vi "dischage_check.vi"(8 "error in":errorcluster) -> (0 "error out":errorcluster)   [LabVIEW 2019]
uses:
  hw-control.ctl
  _ctrl/BP4610_cmd.ctl
  _ctrl/DSP_action.ctl
  _ctrl/init-w-close.ctl
  f7c2fc01-ab73-4381-998f-938b9d5f35cd.vi
  bbb9578e-c01f-4956-a005-e59b9cab9503.vi
  27d873ac-d62a-41d9-9b50-5c3ef5b223c2.vi
  d86a43f2-1348-4437-a8b3-b480884b10c3.vi
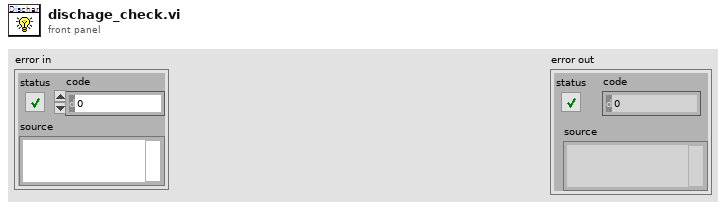
[diagram p1: front panel]
types:
  T1 = typedef "init-w-close.ctl" = enum16{"open", "init", "write", "close"}
  T2 = typedef "DSP_action.ctl" = enum16{"False", "cont", "on", "off", "discont", "protection", "protection_seq", "preread", "level_seq", "level_m", "read", "stop", "exit"}
  T3 = typedef "BP4610_cmd.ctl" = enum16{"open", "read", "set", "set_seq", "limit", "limit_seq", "output on", "output off", "close"}
  T4 = typedef "hw-control.ctl" = enum16{"DL950 ready", "DL950 clear", "DL950 trigger", "DL950 read", "DL950 read seq", "DL950 Tsingle query", "AO 12v", "AO wave", "AO 0v", "relay all-off", "Discharge check", "Discharge", "Relay1", "Relay2", "Relay3", "Relay4", "Relay5", "Relay6", "BP4610 onoff", "BP4610 set", "DSP1500 set", "DSP1500 onoff"}
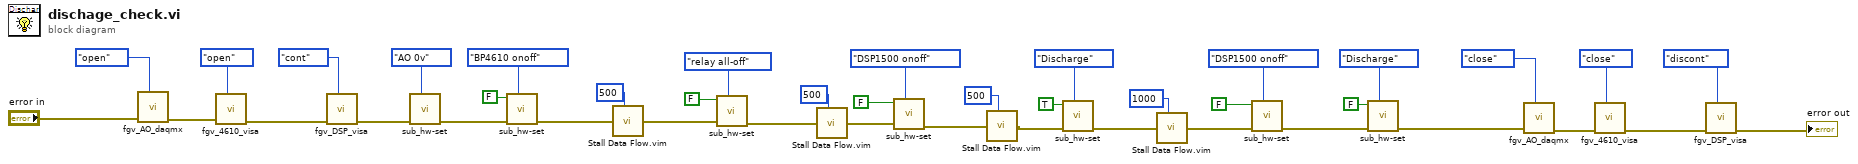
[diagram p0: block diagram]
diagram:
  n1 = call "fgv_AO_daqmx.vi"("cmd"=init-w-close."open", "error in"="error in") -> ("error out"=w9:errorcluster)  [unwired: 9 in]
  n2 = call "fgv_4610_visa.vi"("cmd"=BP4610_cmd."open", "error in"=w9) -> ("error out"=w16:errorcluster)  [unwired: 9 in]
  n3 = call "fgv_DSP_visa.vi"("action"=DSP_action."cont", "error in"=w16) -> ("error out"=w15:errorcluster)  [unwired: 9 in]
  n4 = call "sub_hw-set.vi"("cmd"=hw-control."AO 0v", "error in"=w15) -> ("error out"=w34:errorcluster)  [unwired: 9 in]
  n5 = call "sub_hw-set.vi"("cmd"=hw-control."BP4610 onoff", "error in"=w34, "onoff"=FALSE) -> ("error out"=w2:errorcluster)  [unwired: 8 in]
  n6 = call "Stall Data Flow.vim"("value in"=w2, "milliseconds to wait"=u32 500 ("dt")) -> ("value out"=w1:errorcluster)  [unwired: 1 out]
  n7 = call "sub_hw-set.vi"("cmd"=hw-control."relay all-off", "error in"=w1, "onoff"=FALSE) -> ("error out"=w24:errorcluster)  [unwired: 8 in]
  n8 = call "Stall Data Flow.vim"("value in"=w24, "milliseconds to wait"=u32 500 ("dt")) -> ("value out"=w22:errorcluster)  [unwired: 1 out]
  n9 = call "sub_hw-set.vi"("cmd"=hw-control."DSP1500 onoff", "error in"=w22, "onoff"=FALSE) -> ("error out"=w20:errorcluster)  [unwired: 8 in]
  n10 = call "Stall Data Flow.vim"("value in"=w20, "milliseconds to wait"=u32 500 ("dt")) -> ("value out"=w19:errorcluster)  [unwired: 1 out]
  n11 = call "sub_hw-set.vi"("cmd"=hw-control."Discharge", "error in"=w19, "onoff"=TRUE) -> ("error out"=w32:errorcluster)  [unwired: 8 in]
  n12 = call "Stall Data Flow.vim"("value in"=w32, "milliseconds to wait"=u32 1000 ("dt")) -> ("value out"=w29:errorcluster)  [unwired: 1 out]
  n13 = call "sub_hw-set.vi"("cmd"=hw-control."DSP1500 onoff", "error in"=w29, "onoff"=FALSE) -> ("error out"=w25:errorcluster)  [unwired: 8 in]
  n14 = call "sub_hw-set.vi"("cmd"=hw-control."Discharge", "error in"=w25, "onoff"=FALSE) -> ("error out"=w7:errorcluster)  [unwired: 8 in]
  n15 = call "fgv_AO_daqmx.vi"("cmd"=init-w-close."close", "error in"=w7) -> ("error out"=w6:errorcluster)  [unwired: 9 in]
  n16 = call "fgv_4610_visa.vi"("cmd"=BP4610_cmd."close", "error in"=w6) -> ("error out"=w12:errorcluster)  [unwired: 9 in]
  n17 = call "fgv_DSP_visa.vi"("action"=DSP_action."discont", "error in"=w12) -> ("error out"=→"error out":errorcluster)  [unwired: 9 in]
